vi "NaMCU_configure.vi"() -> ()   [LabVIEW 2020]
uses:
  Instrument drivers/Arduino/ctls_and_globals/Arduino tx msg cluster.ctl
panel:
  in  "DIO 1 mode":u8(ring)=1 items=["Input", "Output"]
  in  "DIO 0 mode":u8(ring)=1 items=["Input", "Output"]
  in  "T1 offset (deg C)":dbl
  in  "T0 offset (deg C)":dbl
  in  "P_atmos offset (Pa)":dbl
  in  "Port":refnum<visa-resource-name>
  in  "Get / Set":u8(ring) items=["Get", "Set"]
  in  "Apply pressure corrections":bool=TRUE
  in  "Tube_D (mm)":dbl=1.0
  in  "Tube_L (mm)":dbl
  out "Read-back":string
  in  "dP offset (Pa)":dbl
  out "Status comment":string
  in  "Address":u8=1
  # "Use this vi to configure the NaMCU pressure transducer node\nThese settings are retained in EEPROM and recalled on power-up."
  # "PN 17/01/2017"
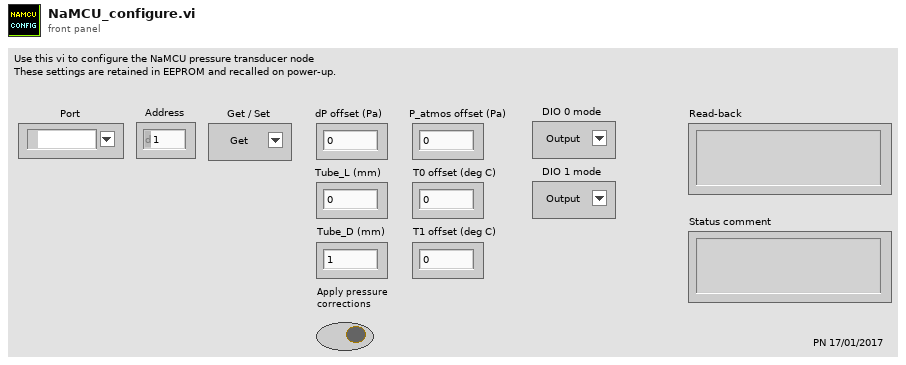
[diagram p1: front panel]
types:
  T1 = typedef "Arduino tx msg cluster.ctl" = cluster{"dest":u8, "A/D/C/I":string, "R/W":string, "chan":u8, "val (float)":sgl}
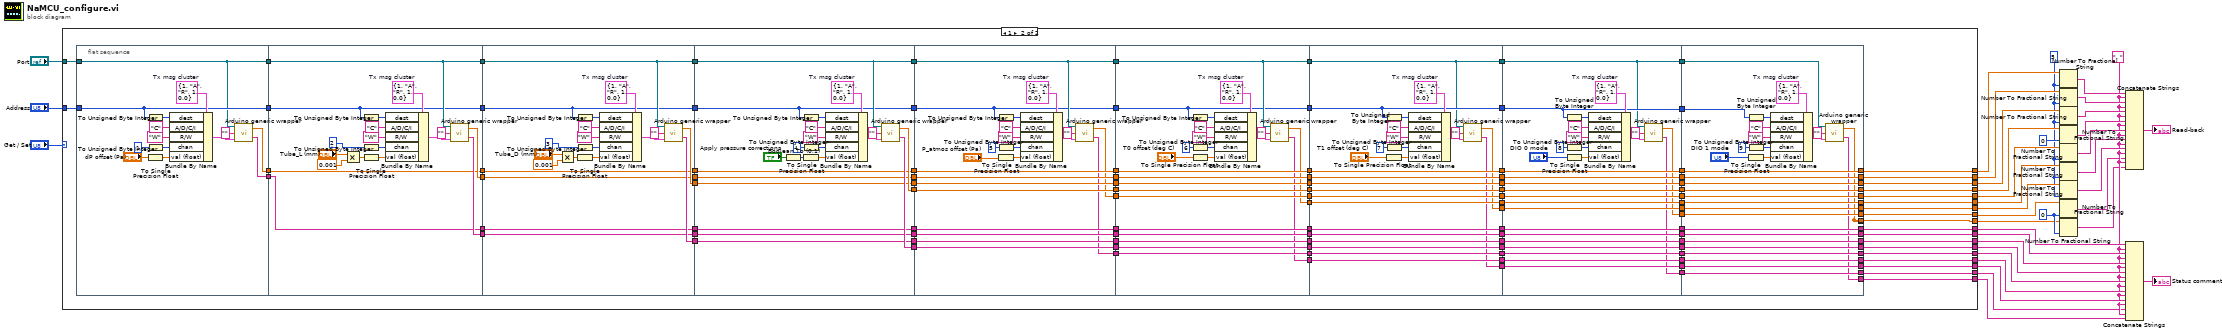
[diagram p0: block diagram]
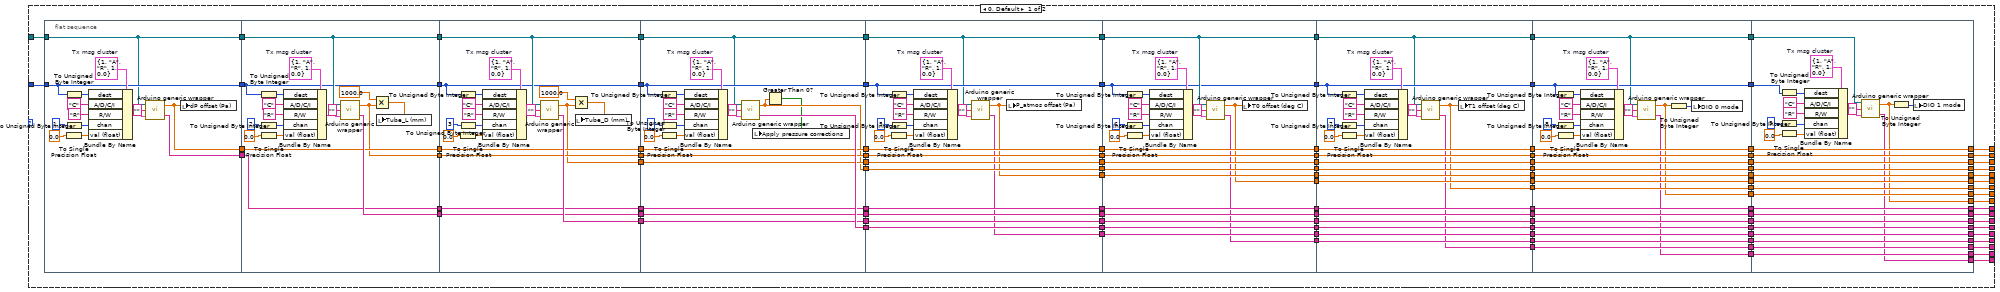
[diagram p2: hidden frame]
diagram:
  w8 = i16 0 ("precision (6)")
  w9 = i16 5 ("precision (6)")
  w7 = ", "
  n1 = case shown="1" "Get / Set" {
    tunnel: "Address" -> [w125 w439]
    tunnel: [w117 w438] -> w31
    tunnel: [w121 w437] -> w30
    tunnel: [w122 w436] -> w28
    tunnel: [w118 w435] -> w27
    tunnel: [w119 w434] -> w26
    tunnel: [w120 w433] -> w25
    tunnel: [w123 w432] -> w24
    tunnel: [w124 w431] -> w23
    tunnel: "Port" -> [w126 w430]
    tunnel: [w84 w419] -> w15
    tunnel: [w78 w405] -> w14
    tunnel: [w75 w389] -> w13
    tunnel: [w82 w418] -> w12
    tunnel: [w79 w404] -> w11
    tunnel: [w76 w388] -> w10
    tunnel: [w43 w356] -> w4
    tunnel: [w42 w354] -> w3
    tunnel: [w38 w351] -> w2
    tunnel: [w37 w350] -> w1
    frame 0, Default {
      n2 = flat-sequence {
        tunnel: w125 -> [w150]
        tunnel: w126 -> [w149]
        tunnel: [w149] -> w144
        tunnel: [w150] -> w143
        tunnel: [w146] -> w142
        tunnel: [w148] -> w141
        tunnel: [w168] -> w140
        tunnel: [w167] -> w139
        tunnel: [w166] -> w138
        tunnel: [w161] -> w137
        tunnel: w144 -> [w168]
        tunnel: w143 -> [w167]
        tunnel: w142 -> [w164]
        tunnel: w141 -> [w165]
        tunnel: [w165] -> w136
        tunnel: [w164] -> w135
        tunnel: w140 -> [w188]
        tunnel: [w188] -> w134
        tunnel: w139 -> [w187]
        tunnel: [w187] -> w133
        tunnel: w138 -> [w185]
        tunnel: w137 -> [w183]
        tunnel: [w186] -> w132
        tunnel: [w179] -> w131
        tunnel: [w185] -> w130
        tunnel: [w184] -> w129
        tunnel: w136 -> [w184]
        tunnel: [w183] -> w128
        tunnel: [w182] -> w127
        tunnel: w135 -> [w182]
        tunnel: w134 -> [w198]
        tunnel: w133 -> [w199]
        tunnel: w132 -> [w207]
        tunnel: w131 -> [w208]
        tunnel: w130 -> [w206]
        tunnel: w129 -> [w205]
        tunnel: w128 -> [w204]
        tunnel: w127 -> [w203]
        tunnel: [w209] -> w116
        tunnel: [w201] -> w115
        tunnel: [w208] -> w114
        tunnel: [w207] -> w113
        tunnel: [w206] -> w112
        tunnel: [w205] -> w111
        tunnel: [w204] -> w110
        tunnel: [w203] -> w109
        tunnel: [w199] -> w92
        tunnel: [w198] -> w91
        tunnel: w116 -> [w239]
        tunnel: w115 -> [w238]
        tunnel: w114 -> [w237]
        tunnel: w113 -> [w236]
        tunnel: w112 -> [w235]
        tunnel: w111 -> [w234]
        tunnel: w110 -> [w233]
        tunnel: w109 -> [w232]
        tunnel: [w239] -> w108
        tunnel: [w238] -> w107
        tunnel: [w237] -> w106
        tunnel: [w236] -> w105
        tunnel: [w235] -> w104
        tunnel: [w234] -> w103
        tunnel: [w233] -> w102
        tunnel: [w232] -> w101
        tunnel: w92 -> [w222]
        tunnel: w91 -> [w221]
        tunnel: [w222] -> w90
        tunnel: [w221] -> w89
        tunnel: [w220] -> w86
        tunnel: [w219] -> w85
        tunnel: w108 -> [w263]
        tunnel: w107 -> [w262]
        tunnel: w106 -> [w261]
        tunnel: w105 -> [w260]
        tunnel: w104 -> [w259]
        tunnel: w103 -> [w258]
        tunnel: w102 -> [w257]
        tunnel: w101 -> [w256]
        tunnel: [w263] -> w100
        tunnel: [w262] -> w99
        tunnel: [w261] -> w98
        tunnel: [w260] -> w97
        tunnel: [w259] -> w96
        tunnel: [w258] -> w95
        tunnel: [w257] -> w94
        tunnel: [w256] -> w93
        tunnel: w90 -> [w243]
        tunnel: w89 -> [w244]
        tunnel: [w243] -> w88
        tunnel: [w244] -> w87
        tunnel: w86 -> [w255]
        tunnel: w85 -> [w254]
        tunnel: [w255] -> w83
        tunnel: [w254] -> w81
        tunnel: [w242] -> w80
        tunnel: [w241] -> w77
        tunnel: w100 -> [w289]
        tunnel: w99 -> [w288]
        tunnel: w98 -> [w287]
        tunnel: w97 -> [w286]
        tunnel: w96 -> [w285]
        tunnel: w95 -> [w284]
        tunnel: w94 -> [w283]
        tunnel: w93 -> [w282]
        tunnel: w88 -> [w266]
        tunnel: w87 -> [w265]
        tunnel: w83 -> [w281]
        tunnel: w81 -> [w280]
        tunnel: w80 -> [w279]
        tunnel: w77 -> [w278]
        tunnel: [w289] -> w74
        tunnel: [w288] -> w73
        tunnel: [w287] -> w72
        tunnel: [w286] -> w71
        tunnel: [w285] -> w70
        tunnel: [w284] -> w69
        tunnel: [w283] -> w68
        tunnel: [w282] -> w67
        tunnel: [w281] -> w66
        tunnel: [w280] -> w65
        tunnel: [w279] -> w64
        tunnel: [w278] -> w63
        tunnel: [w268] -> w62
        tunnel: [w267] -> w61
        tunnel: [w266] -> w46
        tunnel: [w265] -> w45
        tunnel: w74 -> [w318]
        tunnel: w73 -> [w317]
        tunnel: w72 -> [w316]
        tunnel: w71 -> [w315]
        tunnel: w70 -> [w314]
        tunnel: w69 -> [w313]
        tunnel: w68 -> [w312]
        tunnel: w67 -> [w311]
        tunnel: w66 -> [w310]
        tunnel: w65 -> [w309]
        tunnel: w64 -> [w308]
        tunnel: w63 -> [w307]
        tunnel: w62 -> [w306]
        tunnel: w61 -> [w305]
        tunnel: [w318] -> w60
        tunnel: [w317] -> w59
        tunnel: [w316] -> w58
        tunnel: [w315] -> w57
        tunnel: [w314] -> w56
        tunnel: [w313] -> w55
        tunnel: [w312] -> w54
        tunnel: [w311] -> w53
        tunnel: [w310] -> w52
        tunnel: [w309] -> w51
        tunnel: [w308] -> w50
        tunnel: [w307] -> w49
        tunnel: [w306] -> w48
        tunnel: [w305] -> w47
        tunnel: w46 -> [w292]
        tunnel: w45 -> [w291]
        tunnel: [w294] -> w44
        tunnel: [w293] -> w41
        tunnel: [w292] -> w40
        tunnel: [w291] -> w39
        tunnel: [w336] -> w75
        tunnel: [w337] -> w76
        tunnel: [w338] -> w78
        tunnel: [w339] -> w79
        tunnel: [w340] -> w82
        tunnel: [w341] -> w84
        tunnel: [w342] -> w124
        tunnel: [w343] -> w123
        tunnel: [w344] -> w120
        tunnel: [w345] -> w119
        tunnel: [w346] -> w118
        tunnel: [w347] -> w122
        tunnel: [w348] -> w121
        tunnel: [w349] -> w117
        tunnel: w60 -> [w349]
        tunnel: w59 -> [w348]
        tunnel: w58 -> [w347]
        tunnel: w57 -> [w346]
        tunnel: w56 -> [w345]
        tunnel: w55 -> [w344]
        tunnel: w54 -> [w343]
        tunnel: w53 -> [w342]
        tunnel: w52 -> [w341]
        tunnel: w51 -> [w340]
        tunnel: w50 -> [w339]
        tunnel: w49 -> [w338]
        tunnel: w48 -> [w337]
        tunnel: w47 -> [w336]
        tunnel: w44 -> [w335]
        tunnel: [w335] -> w43
        tunnel: [w334] -> w42
        tunnel: w41 -> [w334]
        tunnel: w40 -> [w324]
        tunnel: w39 -> [w323]
        tunnel: [w321] -> w38
        tunnel: [w320] -> w37
        frame #0 {
          w158 = T1 {"dest"=1, "A/D/C/I"="A", "R/W"="R", "chan"=1, "val (float)"=0.0}  # Tx msg cluster
          n3 = To Unsigned Byte Integer(number=w150) -> (unsigned 8bit integer=w156:u8)
          n4 = To Unsigned Byte Integer(number=u8 1) -> (unsigned 8bit integer=w157:u8)
          n5 = To Single Precision Float(number=0.0) -> (single precision float=w154:sgl)
          n6 = Bundle By Name(cluster=w158, "dest"=w156, "A/D/C/I"="C" ("A/D"), "R/W"="R", "chan"=w157, "val (float)"=w154) -> (w155:T1)
          n7 = call "Arduino generic wrapper.vi"("Tx msg cluster"=w155, "Channel Name"="", "Port name"=w149) -> ("Scan comment"=w148:string, "Output"=w146:dbl)
          n8 = local write "dP offset (Pa)"(w146) -> ()
        }
        frame #1 {
          w169 = T1 {"dest"=1, "A/D/C/I"="A", "R/W"="R", "chan"=1, "val (float)"=0.0}  # Tx msg cluster
          n9 = To Unsigned Byte Integer(number=w167) -> (unsigned 8bit integer=w171:u8)
          n10 = To Unsigned Byte Integer(number=u8 2) -> (unsigned 8bit integer=w170:u8)
          n11 = To Single Precision Float(number=0.0) -> (single precision float=w173:sgl)
          n12 = Bundle By Name(cluster=w169, "dest"=w171, "A/D/C/I"="C" ("A/D"), "R/W"="R", "chan"=w170, "val (float)"=w173) -> (w172:T1)
          n13 = call "Arduino generic wrapper.vi"("Tx msg cluster"=w172, "Channel Name"="", "Port name"=w168) -> ("Scan comment"=w166:string, "Output"=w161:dbl)
          n14 = Multiply(x=1000.0 ("y"), y=w161) -> (x*y=w160:dbl)
          n15 = local write "Tube_L (mm)"(w160) -> ()
        }
        frame #2 {
          w196 = T1 {"dest"=1, "A/D/C/I"="A", "R/W"="R", "chan"=1, "val (float)"=0.0}  # Tx msg cluster
          n16 = To Unsigned Byte Integer(number=w187) -> (unsigned 8bit integer=w194:u8)
          n17 = To Unsigned Byte Integer(number=u8 3) -> (unsigned 8bit integer=w195:u8)
          n18 = To Single Precision Float(number=0.0) -> (single precision float=w192:sgl)
          n19 = Bundle By Name(cluster=w196, "dest"=w194, "A/D/C/I"="C" ("A/D"), "R/W"="R", "chan"=w195, "val (float)"=w192) -> (w193:T1)
          n20 = call "Arduino generic wrapper.vi"("Tx msg cluster"=w193, "Channel Name"="", "Port name"=w188) -> ("Scan comment"=w186:string, "Output"=w179:dbl)
          n21 = Multiply(x=1000.0 ("y"), y=w179) -> (x*y=w178:dbl)
          n22 = local write "Tube_D (mm)"(w178) -> ()
        }
        frame #3 {
          w216 = T1 {"dest"=1, "A/D/C/I"="A", "R/W"="R", "chan"=1, "val (float)"=0.0}  # Tx msg cluster
          n23 = To Unsigned Byte Integer(number=w199) -> (unsigned 8bit integer=w210:u8)
          n24 = To Unsigned Byte Integer(number=u8 4) -> (unsigned 8bit integer=w211:u8)
          n25 = To Single Precision Float(number=0.0) -> (single precision float=w213:sgl)
          n26 = Bundle By Name(cluster=w216, "dest"=w210, "A/D/C/I"="C" ("A/D"), "R/W"="R", "chan"=w211, "val (float)"=w213) -> (w212:T1)
          n27 = call "Arduino generic wrapper.vi"("Tx msg cluster"=w212, "Channel Name"="", "Port name"=w198) -> ("Scan comment"=w209:string, "Output"=w201:dbl)
          n28 = Greater Than 0?(x=w201) -> (x > 0?=w200:bool)
          n29 = local write "Apply pressure corrections"(w200) -> ()
        }
        frame #4 {
          w224 = T1 {"dest"=1, "A/D/C/I"="A", "R/W"="R", "chan"=1, "val (float)"=0.0}  # Tx msg cluster
          n30 = To Unsigned Byte Integer(number=w222) -> (unsigned 8bit integer=w230:u8)
          n31 = To Unsigned Byte Integer(number=u8 5) -> (unsigned 8bit integer=w229:u8)
          n32 = To Single Precision Float(number=0.0) -> (single precision float=w227:sgl)
          n33 = Bundle By Name(cluster=w224, "dest"=w230, "A/D/C/I"="C" ("A/D"), "R/W"="R", "chan"=w229, "val (float)"=w227) -> (w228:T1)
          n34 = call "Arduino generic wrapper.vi"("Tx msg cluster"=w228, "Channel Name"="", "Port name"=w221) -> ("Scan comment"=w220:string, "Output"=w219:dbl)
          n35 = local write "P_atmos offset (Pa)"(w219) -> ()
        }
        frame #5 {
          w252 = T1 {"dest"=1, "A/D/C/I"="A", "R/W"="R", "chan"=1, "val (float)"=0.0}  # Tx msg cluster
          n36 = To Unsigned Byte Integer(number=w243) -> (unsigned 8bit integer=w246:u8)
          n37 = To Unsigned Byte Integer(number=u8 6) -> (unsigned 8bit integer=w247:u8)
          n38 = To Single Precision Float(number=0.0) -> (single precision float=w249:sgl)
          n39 = Bundle By Name(cluster=w252, "dest"=w246, "A/D/C/I"="C" ("A/D"), "R/W"="R", "chan"=w247, "val (float)"=w249) -> (w248:T1)
          n40 = call "Arduino generic wrapper.vi"("Tx msg cluster"=w248, "Channel Name"="", "Port name"=w244) -> ("Scan comment"=w241:string, "Output"=w242:dbl)
          n41 = local write "T0 offset (deg C)"(w242) -> ()
        }
        frame #6 {
          w270 = T1 {"dest"=1, "A/D/C/I"="A", "R/W"="R", "chan"=1, "val (float)"=0.0}  # Tx msg cluster
          n42 = To Unsigned Byte Integer(number=w266) -> (unsigned 8bit integer=w276:u8)
          n43 = To Unsigned Byte Integer(number=u8 7) -> (unsigned 8bit integer=w275:u8)
          n44 = To Single Precision Float(number=0.0) -> (single precision float=w273:sgl)
          n45 = Bundle By Name(cluster=w270, "dest"=w276, "A/D/C/I"="C" ("A/D"), "R/W"="R", "chan"=w275, "val (float)"=w273) -> (w274:T1)
          n46 = call "Arduino generic wrapper.vi"("Tx msg cluster"=w274, "Channel Name"="", "Port name"=w265) -> ("Scan comment"=w267:string, "Output"=w268:dbl)
          n47 = local write "T1 offset (deg C)"(w268) -> ()
        }
        frame #7 {
          w303 = T1 {"dest"=1, "A/D/C/I"="A", "R/W"="R", "chan"=1, "val (float)"=0.0}  # Tx msg cluster
          n48 = To Unsigned Byte Integer(number=w292) -> (unsigned 8bit integer=w297:u8)
          n49 = To Unsigned Byte Integer(number=u8 8) -> (unsigned 8bit integer=w298:u8)
          n50 = To Single Precision Float(number=0.0) -> (single precision float=w300:sgl)
          n51 = Bundle By Name(cluster=w303, "dest"=w297, "A/D/C/I"="C" ("A/D"), "R/W"="R", "chan"=w298, "val (float)"=w300) -> (w299:T1)
          n52 = call "Arduino generic wrapper.vi"("Tx msg cluster"=w299, "Channel Name"="", "Port name"=w291) -> ("Scan comment"=w294:string, "Output"=w293:dbl)
          n53 = To Unsigned Byte Integer(number=w293) -> (unsigned 8bit integer=w295:u8)
          n54 = local write "DIO 0 mode"(w295) -> ()
        }
        frame #8 {
          w326 = T1 {"dest"=1, "A/D/C/I"="A", "R/W"="R", "chan"=1, "val (float)"=0.0}  # Tx msg cluster
          n55 = To Unsigned Byte Integer(number=w324) -> (unsigned 8bit integer=w332:u8)
          n56 = To Unsigned Byte Integer(number=u8 9) -> (unsigned 8bit integer=w331:u8)
          n57 = To Single Precision Float(number=0.0) -> (single precision float=w329:sgl)
          n58 = Bundle By Name(cluster=w326, "dest"=w332, "A/D/C/I"="C" ("A/D"), "R/W"="R", "chan"=w331, "val (float)"=w329) -> (w330:T1)
          n59 = call "Arduino generic wrapper.vi"("Tx msg cluster"=w330, "Channel Name"="", "Port name"=w323) -> ("Scan comment"=w321:string, "Output"=w320:dbl)
          n60 = To Unsigned Byte Integer(number=w320) -> (unsigned 8bit integer=w322:u8)
          n61 = local write "DIO 1 mode"(w322) -> ()
        }
      }
    }
    frame 1 {
      n62 = flat-sequence {
        tunnel: w439 -> [w463]
        tunnel: w430 -> [w462]
        tunnel: [w462] -> w457
        tunnel: [w463] -> w456
        tunnel: [w461] -> w455
        tunnel: [w460] -> w454
        tunnel: [w481] -> w453
        tunnel: [w480] -> w452
        tunnel: [w479] -> w451
        tunnel: [w478] -> w450
        tunnel: w457 -> [w481]
        tunnel: w456 -> [w480]
        tunnel: w455 -> [w476]
        tunnel: w454 -> [w477]
        tunnel: [w477] -> w449
        tunnel: [w476] -> w448
        tunnel: w453 -> [w501]
        tunnel: [w501] -> w447
        tunnel: w452 -> [w500]
        tunnel: [w500] -> w446
        tunnel: w451 -> [w497]
        tunnel: w450 -> [w495]
        tunnel: [w499] -> w445
        tunnel: [w498] -> w444
        tunnel: [w497] -> w443
        tunnel: [w496] -> w442
        tunnel: w449 -> [w496]
        tunnel: [w495] -> w441
        tunnel: [w494] -> w440
        tunnel: w448 -> [w494]
        tunnel: w447 -> [w512]
        tunnel: w446 -> [w511]
        tunnel: w445 -> [w517]
        tunnel: w444 -> [w518]
        tunnel: w443 -> [w516]
        tunnel: w442 -> [w515]
        tunnel: w441 -> [w514]
        tunnel: w440 -> [w513]
        tunnel: [w522] -> w429
        tunnel: [w521] -> w428
        tunnel: [w518] -> w427
        tunnel: [w517] -> w426
        tunnel: [w516] -> w425
        tunnel: [w515] -> w424
        tunnel: [w514] -> w423
        tunnel: [w513] -> w422
        tunnel: [w512] -> w421
        tunnel: [w511] -> w420
        tunnel: w429 -> [w552]
        tunnel: w428 -> [w551]
        tunnel: w427 -> [w550]
        tunnel: w426 -> [w549]
        tunnel: w425 -> [w548]
        tunnel: w424 -> [w547]
        tunnel: w423 -> [w546]
        tunnel: w422 -> [w545]
        tunnel: w421 -> [w533]
        tunnel: w420 -> [w532]
        tunnel: [w552] -> w417
        tunnel: [w551] -> w416
        tunnel: [w550] -> w415
        tunnel: [w549] -> w414
        tunnel: [w548] -> w413
        tunnel: [w547] -> w412
        tunnel: [w546] -> w411
        tunnel: [w545] -> w410
        tunnel: [w535] -> w409
        tunnel: [w534] -> w408
        tunnel: [w533] -> w407
        tunnel: [w532] -> w406
        tunnel: w417 -> [w576]
        tunnel: w416 -> [w575]
        tunnel: w415 -> [w574]
        tunnel: w414 -> [w573]
        tunnel: w413 -> [w572]
        tunnel: w412 -> [w571]
        tunnel: w411 -> [w570]
        tunnel: w410 -> [w569]
        tunnel: w409 -> [w568]
        tunnel: w408 -> [w567]
        tunnel: w407 -> [w555]
        tunnel: w406 -> [w554]
        tunnel: [w576] -> w403
        tunnel: [w575] -> w402
        tunnel: [w574] -> w401
        tunnel: [w573] -> w400
        tunnel: [w572] -> w399
        tunnel: [w571] -> w398
        tunnel: [w570] -> w397
        tunnel: [w569] -> w396
        tunnel: [w568] -> w395
        tunnel: [w567] -> w394
        tunnel: [w557] -> w393
        tunnel: [w556] -> w392
        tunnel: [w555] -> w391
        tunnel: [w554] -> w390
        tunnel: w403 -> [w602]
        tunnel: w402 -> [w601]
        tunnel: w401 -> [w600]
        tunnel: w400 -> [w599]
        tunnel: w399 -> [w598]
        tunnel: w398 -> [w597]
        tunnel: w397 -> [w596]
        tunnel: w396 -> [w595]
        tunnel: w395 -> [w594]
        tunnel: w394 -> [w593]
        tunnel: w393 -> [w592]
        tunnel: w392 -> [w591]
        tunnel: w391 -> [w578]
        tunnel: w390 -> [w579]
        tunnel: [w602] -> w387
        tunnel: [w601] -> w386
        tunnel: [w600] -> w385
        tunnel: [w599] -> w384
        tunnel: [w598] -> w383
        tunnel: [w597] -> w382
        tunnel: [w596] -> w381
        tunnel: [w595] -> w380
        tunnel: [w594] -> w379
        tunnel: [w593] -> w378
        tunnel: [w592] -> w377
        tunnel: [w591] -> w376
        tunnel: [w581] -> w375
        tunnel: [w580] -> w374
        tunnel: [w579] -> w359
        tunnel: [w578] -> w358
        tunnel: w387 -> [w630]
        tunnel: w386 -> [w629]
        tunnel: w385 -> [w628]
        tunnel: w384 -> [w627]
        tunnel: w383 -> [w626]
        tunnel: w382 -> [w625]
        tunnel: w381 -> [w624]
        tunnel: w380 -> [w623]
        tunnel: w379 -> [w622]
        tunnel: w378 -> [w621]
        tunnel: w377 -> [w620]
        tunnel: w376 -> [w619]
        tunnel: w375 -> [w618]
        tunnel: w374 -> [w617]
        tunnel: [w630] -> w373
        tunnel: [w629] -> w372
        tunnel: [w628] -> w371
        tunnel: [w627] -> w370
        tunnel: [w626] -> w369
        tunnel: [w625] -> w368
        tunnel: [w624] -> w367
        tunnel: [w623] -> w366
        tunnel: [w622] -> w365
        tunnel: [w621] -> w364
        tunnel: [w620] -> w363
        tunnel: [w619] -> w362
        tunnel: [w618] -> w361
        tunnel: [w617] -> w360
        tunnel: w359 -> [w605]
        tunnel: w358 -> [w604]
        tunnel: [w607] -> w357
        tunnel: [w606] -> w355
        tunnel: [w605] -> w353
        tunnel: [w604] -> w352
        tunnel: [w647] -> w388
        tunnel: [w648] -> w389
        tunnel: [w649] -> w404
        tunnel: [w650] -> w405
        tunnel: [w651] -> w418
        tunnel: [w652] -> w419
        tunnel: [w653] -> w431
        tunnel: [w654] -> w432
        tunnel: [w655] -> w433
        tunnel: [w656] -> w434
        tunnel: [w657] -> w435
        tunnel: [w658] -> w436
        tunnel: [w659] -> w437
        tunnel: [w660] -> w438
        tunnel: w373 -> [w660]
        tunnel: w372 -> [w659]
        tunnel: w371 -> [w658]
        tunnel: w370 -> [w657]
        tunnel: w369 -> [w656]
        tunnel: w368 -> [w655]
        tunnel: w367 -> [w654]
        tunnel: w366 -> [w653]
        tunnel: w365 -> [w652]
        tunnel: w364 -> [w651]
        tunnel: w363 -> [w650]
        tunnel: w362 -> [w649]
        tunnel: w361 -> [w648]
        tunnel: w360 -> [w647]
        tunnel: w357 -> [w646]
        tunnel: [w646] -> w356
        tunnel: w355 -> [w645]
        tunnel: [w645] -> w354
        tunnel: w353 -> [w636]
        tunnel: w352 -> [w635]
        tunnel: [w633] -> w351
        tunnel: [w632] -> _
        tunnel: [w632] -> w350
        frame #0 {
          w471 = T1 {"dest"=1, "A/D/C/I"="A", "R/W"="R", "chan"=1, "val (float)"=0.0}  # Tx msg cluster
          n63 = To Unsigned Byte Integer(number=w463) -> (unsigned 8bit integer=w469:u8)
          n64 = To Unsigned Byte Integer(number=u8 1) -> (unsigned 8bit integer=w470:u8)
          n65 = To Single Precision Float(number="dP offset (Pa)") -> (single precision float=w467:sgl)
          n66 = Bundle By Name(cluster=w471, "dest"=w469, "A/D/C/I"="C" ("A/D"), "R/W"="W", "chan"=w470, "val (float)"=w467) -> (w468:T1)
          n67 = call "Arduino generic wrapper.vi"("Tx msg cluster"=w468, "Channel Name"="", "Port name"=w462) -> ("Scan comment"=w460:string, "Output"=w461:dbl)
        }
        frame #1 {
          w482 = T1 {"dest"=1, "A/D/C/I"="A", "R/W"="R", "chan"=1, "val (float)"=0.0}  # Tx msg cluster
          n68 = Multiply(x="Tube_L (mm)", y=0.001) -> (x*y=w474:dbl)
          n69 = To Unsigned Byte Integer(number=w480) -> (unsigned 8bit integer=w484:u8)
          n70 = To Unsigned Byte Integer(number=u8 2) -> (unsigned 8bit integer=w483:u8)
          n71 = To Single Precision Float(number=w474) -> (single precision float=w486:sgl)
          n72 = Bundle By Name(cluster=w482, "dest"=w484, "A/D/C/I"="C" ("A/D"), "R/W"="W", "chan"=w483, "val (float)"=w486) -> (w485:T1)
          n73 = call "Arduino generic wrapper.vi"("Tx msg cluster"=w485, "Channel Name"="", "Port name"=w481) -> ("Scan comment"=w479:string, "Output"=w478:dbl)
        }
        frame #2 {
          w509 = T1 {"dest"=1, "A/D/C/I"="A", "R/W"="R", "chan"=1, "val (float)"=0.0}  # Tx msg cluster
          n74 = Multiply(x="Tube_D (mm)", y=0.001) -> (x*y=w491:dbl)
          n75 = To Unsigned Byte Integer(number=w500) -> (unsigned 8bit integer=w507:u8)
          n76 = To Unsigned Byte Integer(number=u8 3) -> (unsigned 8bit integer=w508:u8)
          n77 = To Single Precision Float(number=w491) -> (single precision float=w505:sgl)
          n78 = Bundle By Name(cluster=w509, "dest"=w507, "A/D/C/I"="C" ("A/D"), "R/W"="W", "chan"=w508, "val (float)"=w505) -> (w506:T1)
          n79 = call "Arduino generic wrapper.vi"("Tx msg cluster"=w506, "Channel Name"="", "Port name"=w501) -> ("Scan comment"=w499:string, "Output"=w498:dbl)
        }
        frame #3 {
          w529 = T1 {"dest"=1, "A/D/C/I"="A", "R/W"="R", "chan"=1, "val (float)"=0.0}  # Tx msg cluster
          n80 = Boolean To (0,1)(Boolean="Apply pressure corrections") -> (0, 1=w519:i16)
          n81 = To Unsigned Byte Integer(number=w511) -> (unsigned 8bit integer=w523:u8)
          n82 = To Unsigned Byte Integer(number=u8 4) -> (unsigned 8bit integer=w524:u8)
          n83 = To Single Precision Float(number=w519) -> (single precision float=w526:sgl)
          n84 = Bundle By Name(cluster=w529, "dest"=w523, "A/D/C/I"="C" ("A/D"), "R/W"="W", "chan"=w524, "val (float)"=w526) -> (w525:T1)
          n85 = call "Arduino generic wrapper.vi"("Tx msg cluster"=w525, "Channel Name"="", "Port name"=w512) -> ("Scan comment"=w522:string, "Output"=w521:dbl)
        }
        frame #4 {
          w538 = T1 {"dest"=1, "A/D/C/I"="A", "R/W"="R", "chan"=1, "val (float)"=0.0}  # Tx msg cluster
          n86 = To Unsigned Byte Integer(number=w532) -> (unsigned 8bit integer=w544:u8)
          n87 = To Unsigned Byte Integer(number=u8 5) -> (unsigned 8bit integer=w543:u8)
          n88 = To Single Precision Float(number="P_atmos offset (Pa)") -> (single precision float=w541:sgl)
          n89 = Bundle By Name(cluster=w538, "dest"=w544, "A/D/C/I"="C" ("A/D"), "R/W"="W", "chan"=w543, "val (float)"=w541) -> (w542:T1)
          n90 = call "Arduino generic wrapper.vi"("Tx msg cluster"=w542, "Channel Name"="", "Port name"=w533) -> ("Scan comment"=w535:string, "Output"=w534:dbl)
        }
        frame #5 {
          w565 = T1 {"dest"=1, "A/D/C/I"="A", "R/W"="R", "chan"=1, "val (float)"=0.0}  # Tx msg cluster
          n91 = To Unsigned Byte Integer(number=w554) -> (unsigned 8bit integer=w559:u8)
          n92 = To Unsigned Byte Integer(number=u8 6) -> (unsigned 8bit integer=w560:u8)
          n93 = To Single Precision Float(number="T0 offset (deg C)") -> (single precision float=w562:sgl)
          n94 = Bundle By Name(cluster=w565, "dest"=w559, "A/D/C/I"="C" ("A/D"), "R/W"="W", "chan"=w560, "val (float)"=w562) -> (w561:T1)
          n95 = call "Arduino generic wrapper.vi"("Tx msg cluster"=w561, "Channel Name"="", "Port name"=w555) -> ("Scan comment"=w557:string, "Output"=w556:dbl)
        }
        frame #6 {
          w584 = T1 {"dest"=1, "A/D/C/I"="A", "R/W"="R", "chan"=1, "val (float)"=0.0}  # Tx msg cluster
          n96 = To Unsigned Byte Integer(number=w579) -> (unsigned 8bit integer=w590:u8)
          n97 = To Unsigned Byte Integer(number=u8 7) -> (unsigned 8bit integer=w589:u8)
          n98 = To Single Precision Float(number="T1 offset (deg C)") -> (single precision float=w587:sgl)
          n99 = Bundle By Name(cluster=w584, "dest"=w590, "A/D/C/I"="C" ("A/D"), "R/W"="W", "chan"=w589, "val (float)"=w587) -> (w588:T1)
          n100 = call "Arduino generic wrapper.vi"("Tx msg cluster"=w588, "Channel Name"="", "Port name"=w578) -> ("Scan comment"=w581:string, "Output"=w580:dbl)
        }
        frame #7 {
          w615 = T1 {"dest"=1, "A/D/C/I"="A", "R/W"="R", "chan"=1, "val (float)"=0.0}  # Tx msg cluster
          n101 = To Unsigned Byte Integer(number=w605) -> (unsigned 8bit integer=w609:u8)
          n102 = To Unsigned Byte Integer(number=u8 8) -> (unsigned 8bit integer=w610:u8)
          n103 = To Single Precision Float(number="DIO 0 mode") -> (single precision float=w612:sgl)
          n104 = Bundle By Name(cluster=w615, "dest"=w609, "A/D/C/I"="C" ("A/D"), "R/W"="W", "chan"=w610, "val (float)"=w612) -> (w611:T1)
          n105 = call "Arduino generic wrapper.vi"("Tx msg cluster"=w611, "Channel Name"="", "Port name"=w604) -> ("Scan comment"=w607:string, "Output"=w606:dbl)
        }
        frame #8 {
          w638 = T1 {"dest"=1, "A/D/C/I"="A", "R/W"="R", "chan"=1, "val (float)"=0.0}  # Tx msg cluster
          n106 = To Unsigned Byte Integer(number=w636) -> (unsigned 8bit integer=w644:u8)
          n107 = To Unsigned Byte Integer(number=u8 9) -> (unsigned 8bit integer=w643:u8)
          n108 = To Single Precision Float(number="DIO 1 mode") -> (single precision float=w641:sgl)
          n109 = Bundle By Name(cluster=w638, "dest"=w644, "A/D/C/I"="C" ("A/D"), "R/W"="W", "chan"=w643, "val (float)"=w641) -> (w642:T1)
          n110 = call "Arduino generic wrapper.vi"("Tx msg cluster"=w642, "Channel Name"="", "Port name"=w635) -> ("Scan comment"=w633:string, "Output"=w632:dbl)
        }
      }
    }
  }
  n111 = Number To Fractional String(number=w23, precision (6)=w9) -> (F-format string=w35:string)  [unwired: 2 in]
  n112 = Number To Fractional String(number=w24, precision (6)=w9) -> (F-format string=w34:string)  [unwired: 2 in]
  n113 = Number To Fractional String(number=w28, precision (6)=w9) -> (F-format string=w22:string)  [unwired: 2 in]
  n114 = Number To Fractional String(number=w30, precision (6)=i16 0) -> (F-format string=w21:string)  [unwired: 2 in]
  n115 = Number To Fractional String(number=w12, precision (6)=w9) -> (F-format string=w18:string)  [unwired: 2 in]
  n116 = Number To Fractional String(number=w11, precision (6)=w9) -> (F-format string=w17:string)  [unwired: 2 in]
  n117 = Number To Fractional String(number=w10, precision (6)=w9) -> (F-format string=w16:string)  [unwired: 2 in]
  n118 = Number To Fractional String(number=w3, precision (6)=w8) -> (F-format string=w5:string)  [unwired: 2 in]
  n119 = Number To Fractional String(number=w1, precision (6)=w8) -> (F-format string=w6:string)  [unwired: 2 in]
  n120 = Concatenate Strings(w35, w7, w34, w7, w22, w7, w21, w7, w18, w7, w17, w7, w16, w7, w5, w7, w6) -> (→"Read-back":string)
  n121 = Concatenate Strings(w25, w7, w26, w7, w27, w7, w31, w7, w15, w7, w14, w7, w13, w7, w4, w7, w2) -> (→"Status comment":string)
